vi "ExposeToObjectMap.vi"(8 "BaseName":string, 9 "Skip Parent Name (t)":bool=TRUE, 11 "Value":variant) -> (3 "Object map":T1[](array[typedef]))   [LabVIEW 2017]
uses:
  ExposeObjectMapNamepathData.ctl
  ExposeObjectMapDataTypeEnum.ctl
  ExposeObjectMapContainerTypeEnum.ctl
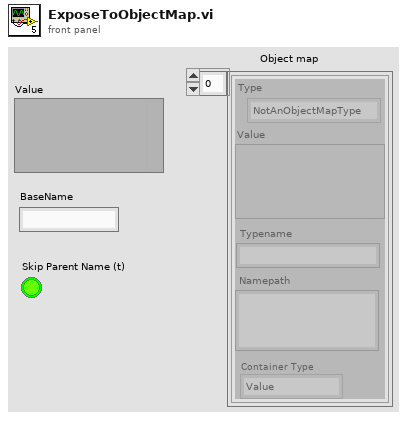
[diagram p1: front panel]
types:
  T1 = typedef "ExposeObjectMapNamepathData.ctl" = cluster{"Type":T2, "Value":variant, "Namepath":string, "Typename":string, "Container Type":T3}
  T2 = typedef "ExposeObjectMapDataTypeEnum.ctl" = enum16{"NotAnObjectMapType", "Real", "Complex", "String", "Boolean"}
  T3 = typedef "ExposeObjectMapContainerTypeEnum.ctl" = enum16{"Value", "Array", "Waveform"}
  T4 = typedef "NI_Data Type.lvlib/Data Type.ctl" = enum8{"Invalid Type", "Void", "I8", "I16", "I32", "I64", "U8", "U16", "U32", "U64", "Single Float", "Double Float", "Extended Float", "Single Complex", "Double Complex", "Extended Complex", "Enum U8", "Enum U16", "Enum U32", "Enum U64", "Single Float With Unit", "Double Float With Unit", "Extended Float With Unit", "Single Complex with Unit", "Double Complex with Unit", "Extended Complex with Unit", "Boolean", "String", "Path", "Picture", "Tag", "Array", "Cluster", "Variant", "LV Variant", "Waveform", "Timestamp", "Digital Waveform", "Digital Data", "ExpressData", "Refnum", "External Data", "VI", "Poly VI", "LabVIEW Class Instance", "Fixed Point"}
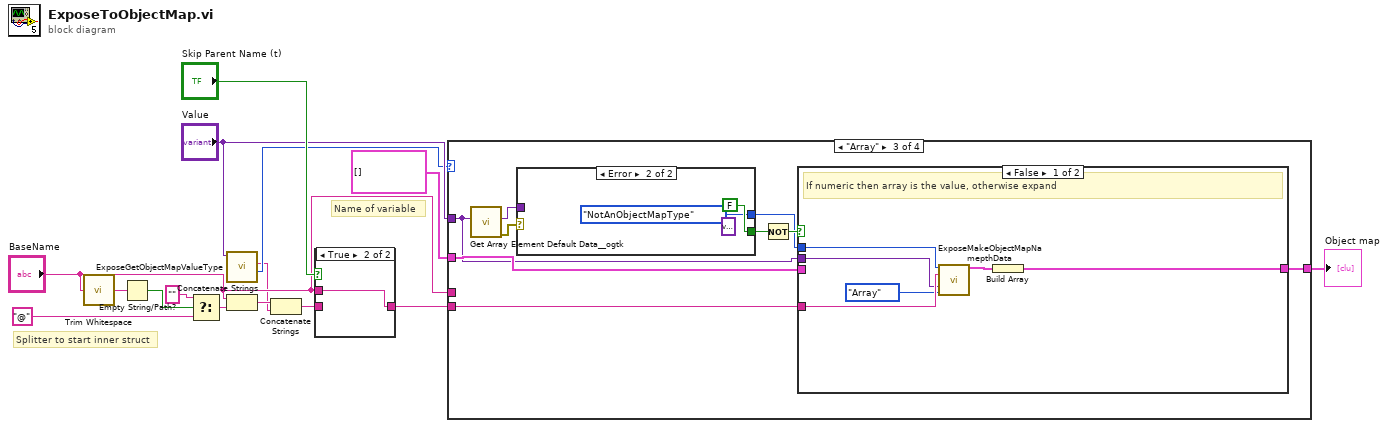
[diagram p0: block diagram]
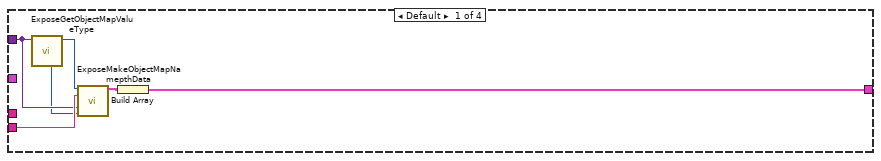
[diagram p3: hidden frame]
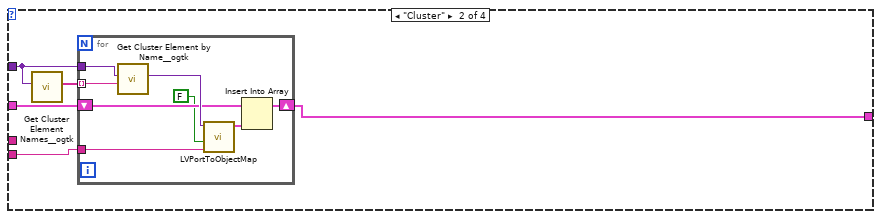
[diagram p4: hidden frame]
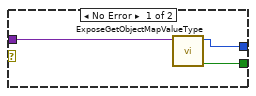
[diagram p5: hidden frame]
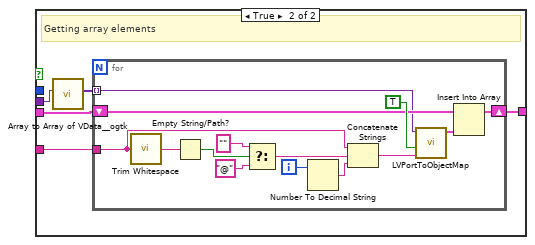
[diagram p6: hidden frame]
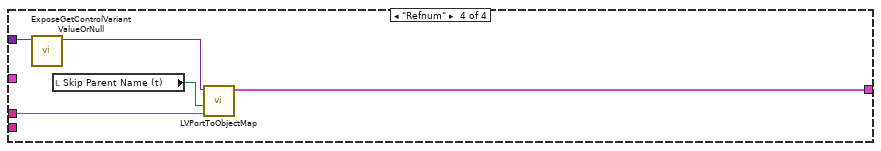
[diagram p7: hidden frame]
diagram:
  # "Splitter to start inner struct"
  # "Name of variable"
  n1 = call <vilib>:"Trim Whitespace.vi"("string"="BaseName") -> ("trimmed string"=w8:string)  [unwired: 1 in]
  n2 = Empty String/Path?(string/path=w8) -> (empty?=w7:bool)
  n3 = Select(t="" ("name"), s=w7, f="@" ("name")) -> (s? t:f=w15:string)
  n4 = call "ExposeGetObjectMapValueType.vi"("Value"="Value") -> ("Type"=w2:T4, "Name"=w1:string)  [unwired: 6 in, 3 out]
  n5 = Concatenate Strings("BaseName", w15) -> (w9:string)
  n6 = Concatenate Strings(w9, w1) -> (w11:string)
  n7 = case shown="True" "Skip Parent Name (t)" {
    tunnel: [w16 w17] -> w12
    tunnel: w11 -> [w16 _]
    tunnel: "BaseName" -> [_ w17]
    frame False {
    }
    frame True {
    }
  }
  n8 = case shown="\"Array\"" w2 {
    tunnel: [w22 w28 w45 w78] -> w5
    tunnel: w12 -> [w20 w27 w42 _]
    tunnel: "BaseName" -> [_ _ _ w79]
    tunnel: T1[] [] -> [_ w25 w41 _]
    tunnel: "Value" -> [w19 w24 w40 w77]
    frame Default {
      n9 = call "ExposeGetObjectMapValueType.vi"("Value"=w19) -> ("ObjectMapType"=w21:T2, "Container Type (Labview Value type)"=w18:T3)  [unwired: 6 in, 3 out]
      n10 = call "ExposeMakeObjectMapNamepthData.vi"("ObjectMapType"=w21, "namepath"=w20, "value"=w19, "Labview Contriner type"=w18) -> ("MatlabDataBundle"=w23:T1)  [unwired: 11 in]
      n11 = Build Array(w23) -> (w22:T1[])
    }
    frame "Cluster" {
      n12 = call <userlib>:"Get Cluster Element Names__ogtk.vi"("Cluster"=w24) -> ("Element Names"=w26:string[])  [unwired: 9 in, 1 out]
      n13 = for {
        shift-right: [w36] -> w28
        shift-left: w25 -> [w32]
        tunnel: w27 -> [w35]
        tunnel: w26 -> [w34] mode=indexing
        tunnel: w24 -> [w30]
        n14 = call <userlib>:"Get Cluster Element by Name__ogtk.vi"("Element Name"=w34, "Cluster"=w30) -> ("VElement"=w33:variant)  [unwired: 7 in, 2 out]
        n15 = call "LVPortToObjectMap.vi"("BaseName"=w35, "Skip Parent Name (t)"=FALSE ("IgnoreContainerName"), "Value"=w33) -> ("Object map"=w31:T1[])  [unwired: 8 in]
        n16 = Insert Into Array(array=w32, new element=w31) -> (w36:T1[])  [unwired: 1 in]
      }
    }
    frame "Array" {
      n17 = call <userlib>:"Get Array Element Default Data__ogtk.vi"("Array"=w40) -> ("error out"=w39:errorcluster, "Array Element Default Data"=w37:variant)  [unwired: 9 in]
      n18 = case shown="Error" w39 {
        tunnel: [w48 FALSE ("IsNumeric")] -> w44
        tunnel: [w47 ExposeObjectMapDataTypeEnum."NotAnObjectMapType" ("MatlabType")] -> w38
        tunnel: w37 -> [w46 _]
        frame No Error {
          n19 = call "ExposeGetObjectMapValueType.vi"("Value"=w46) -> ("IsNumeric"=w48:bool, "ObjectMapType"=w47:T2)  [unwired: 6 in, 3 out]
        }
        frame Error {
          (unwired) variant
        }
      }
      n20 = Not(x=w44) -> (.not. x?=w43:bool)
      n21 = case shown="False" w43 {
        tunnel: [w54 w61] -> w45
        tunnel: w42 -> [w56 w60]
        tunnel: w41 -> [_ w59]
        tunnel: w40 -> [w53 w58]
        tunnel: w38 -> [w52 _]
        frame False {
          # "If numeric then array is the value, otherwise expand"
          n22 = call "ExposeMakeObjectMapNamepthData.vi"("ObjectMapType"=w52, "namepath"=w56, "value"=w53, "Labview Contriner type"=ExposeObjectMapContainerTypeEnum."Array") -> ("MatlabDataBundle"=w55:T1)  [unwired: 11 in]
          n23 = Build Array(w55) -> (w54:T1[])
        }
        frame True {
          # "Getting array elements"
          n24 = call <userlib>:"Array to Array of VData__ogtk.vi"("MultiD Array"=w58) -> ("1D Array of Variants"=w57:variant[])  [unwired: 9 in, 1 out]
          n25 = for {
            shift-right: [w75] -> w61
            shift-left: w59 -> [w71]
            tunnel: w60 -> [w66]
            tunnel: w57 -> [w68] mode=indexing
            i -> [w69]
            n26 = call <vilib>:"Trim Whitespace.vi"("string"=w66) -> ("trimmed string"=w67:string)  [unwired: 1 in]
            n27 = Empty String/Path?(string/path=w67) -> (empty?=w65:bool)
            n28 = Select(t="", s=w65, f="@" ("string")) -> (s? t:f=w62:string)
            n29 = Number To Decimal String(number=w69) -> (decimal integer string=w74:string)  [unwired: 1 in]
            n30 = Concatenate Strings(w66, w62, w74) -> (w73:string)
            n31 = call "LVPortToObjectMap.vi"("BaseName"=w73, "Skip Parent Name (t)"=TRUE ("IgnoreContainerName"), "Value"=w68) -> ("Object map"=w70:T1[])  [unwired: 8 in]
            n32 = Insert Into Array(array=w71, new element=w70) -> (w75:T1[])  [unwired: 1 in]
          }
        }
      }
    }
    frame "Refnum" {
      n33 = call "ExposeGetControlVariantValueOrNull.vi"("ControlVariant"=w77) -> ("Value"=w80:variant)  [unwired: 9 in, 1 out]
      n34 = local read "Skip Parent Name (t)"() -> (w76:bool)
      n35 = call "LVPortToObjectMap.vi"("BaseName"=w79, "Skip Parent Name (t)"=w76, "Value"=w80) -> ("Object map"=w78:T1[])  [unwired: 8 in]
    }
  }
  "Object map" <- w5
